vi "Save Configuration.vi"(8 "error in (no error)":errorcluster, 10 "File path":path, 11 "Measure Object in":refnum<class "Template Module.lvclass">) -> (0 "error out":errorcluster, 1 "Section out":string, 2 "File path out":path, 3 "Measure Object out":refnum<class "Template Module.lvclass">)   [LabVIEW 2016, in "Template Module.lvclass"]
uses:
  Template Module.lvclass
  Template Module.lvclass/Template Module.ctl
  Template Module Messages/Save Configuration Msg/Save Configuration Msg.lvclass/Save Configuration Msg.ctl
  <vilib>/ActorFramework/Message Enqueuer/Message Enqueuer.lvclass/Message Enqueuer.ctl
  Read Name.vi
  <vilib>/ActorFramework/Message Enqueuer/Enqueue.vi
  Template Module Messages/Save Configuration Msg/Save Configuration Msg.lvclass
  C:/Program Files (x86)/National Instruments/LabVIEW 2016/vi.lib/ActorFramework/Message/Message.lvclass
  <vilib>/ActorFramework/Message Priority Queue/Priority Enqueue.vi
panel:
  out "Object names":string[](array[string])
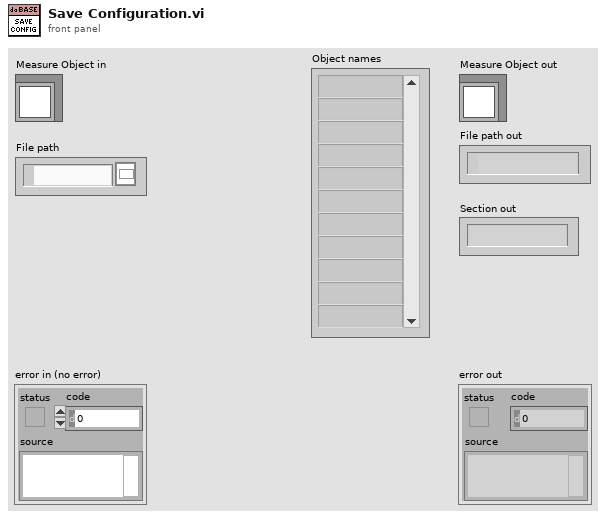
[diagram p1: front panel]
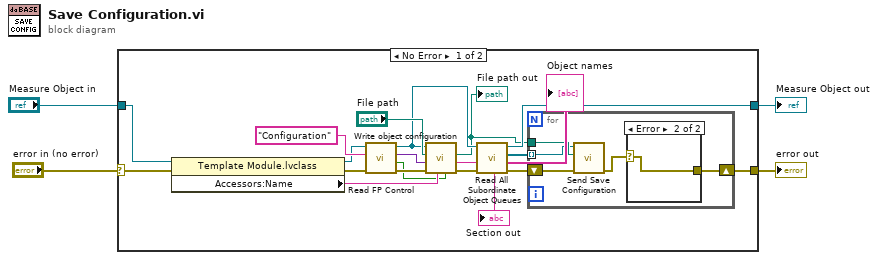
[diagram p0: block diagram]
diagram:
  n1 = case shown="No Error" "error in (no error)" {
    selector: "error in (no error)" -> [w18 w32]
    tunnel: [w11 w32] -> w3
    tunnel: [w12 w31] -> w1
    tunnel: "Measure Object in" -> [w17 w31]
    frame No Error {
      n2 = property class="Template Module.lvclass"(reference=w17, error in=w18) -> (reference out=w16:refnum<class "Template Module.lvclass">, error out=w19:errorcluster, "Accessors:Name"=w22:string)
      n3 = call-dynamic "Read FP Control.vi"("error in (no error)"=w19, "Control Name"="Configuration", "Measure Object in"=w16) -> ("error out"=w10:errorcluster, "Present"=w5:bool, "Control Value"=w21:variant, "Measure Object out"=w13:refnum<class "Template Module.lvclass">)  [unwired: 5 in]
      n4 = call "Write object configuration.vi"("Present"=w5, "Object name"=w22, "Error In"=w10, "Configuration"=w21, "File path"="File path", "object"=w13) -> ("Error Out"=w9:errorcluster, "Section out"=→"Section out":string, "File path out"=w8:path)  [unwired: 3 in]
      "File path out" <- w8
      n5 = call-dynamic "Read All Subordinate Object Queues.vi"("error in (no error)"=w9, "Measure Object in"=w13) -> ("error out"=w14:errorcluster, "Object names"=→"Object names":string[], "Object enqueuers"=w15:refnum<class "Message Enqueuer.lvclass">[], "Measure Object out"=w12:refnum<class "Template Module.lvclass">)  [unwired: 6 in]
      n6 = for {
        tunnel: w8 -> [w28]
        tunnel: w15 -> [w27] mode=indexing
        shift-right: [w24] -> w11
        shift-left: w14 -> [w26]
        n7 = call "Send Save Configuration.vi"("error in (no error)"=w26, "File path"=w28, "Message Enqueuer"=w27) -> ("error out"=w25:errorcluster)  [unwired: 7 in, 1 out]
        n8 = case shown="Error" w25 {
          selector: w25 -> [w29 w30]
          tunnel: [w29 w30] -> w24
          frame No Error {
          }
          frame Error {
          }
        }
      }
    }
    frame Error {
    }
  }
  "error out" <- w3
  "Measure Object out" <- w1
